vi "Update UI.vi"(7 "This VI":refnum<vi>, 8 "error in (no error)":errorcluster, 11 "Application in":refnum<class "Application.lvclass">) -> (0 "error out":errorcluster, 1 "Time":u32, 3 "Application out":refnum<class "Application.lvclass">)   [LabVIEW 2021, in "Application.lvclass"]
uses:
  Application.lvclass
  Application.lvclass/Application.ctl
  Board Game_class/Board Game.lvclass
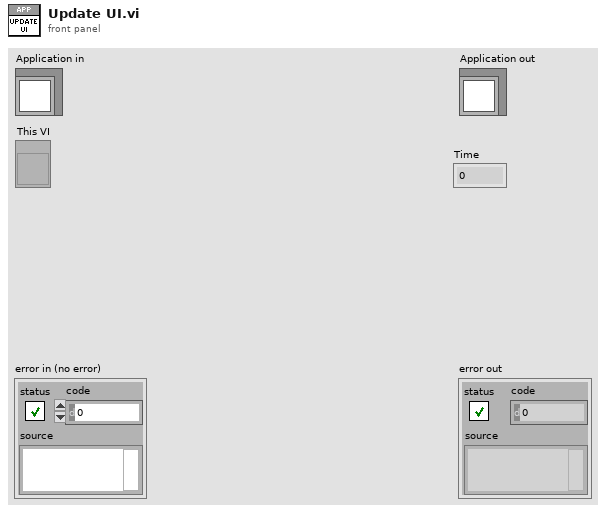
[diagram p1: front panel]
types:
  T1 = typedef "Application.lvclass/Packed Refs.ctl" = cluster{"graphics queue":refnum<queue>, "Pause Game Event":refnum<user-event>, "Stop Control Loop":refnum<user-event>, "Direction":refnum<notifier>, "play sound":refnum<user-event>, "stop sound":refnum<user-event>, "Timer":refnum<data-value>}
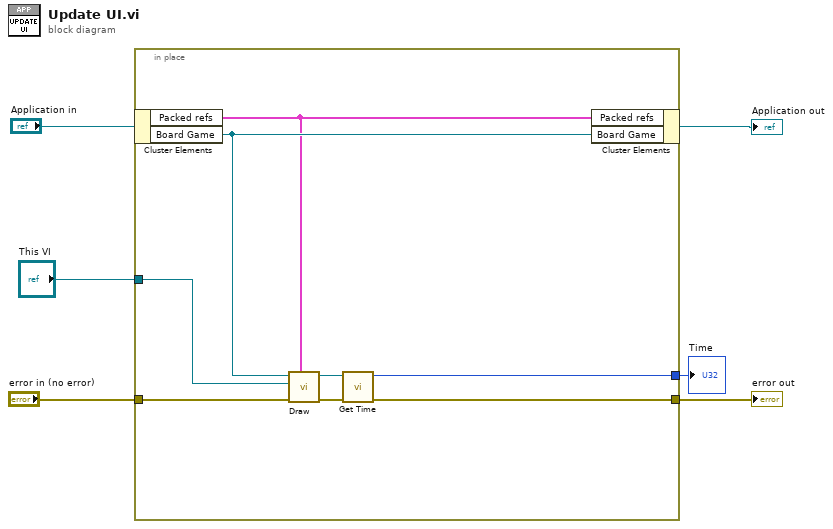
[diagram p0: block diagram]
diagram:
  n1 = in-place {
    in-place-border: "error in (no error)" -> [w13]
    in-place-border: [w11] -> w4
    in-place-border: "This VI" -> [w8]
    in-place-border: [w7] -> w1
    n2 = in-place-cluster #1("Application in") -> ("Packed refs"=w9:T1, "Board Game"=w10:refnum<class "Board Game.lvclass">)
    n3 = call "Draw.vi"("Packed refs"=w9, "error in (no error)"=w13, "This VI"=w8, "Board Game in"=w10) -> ("error out"=w12:errorcluster, "Board Game out"=w14:refnum<class "Board Game.lvclass">)  [unwired: 6 in]
    n4 = call "Get Time.vi"("error in (no error)"=w12, "Board Game in"=w14) -> ("error out"=w11:errorcluster, "Time"=w7:u32)  [unwired: 8 in]
    n5 = in-place-cluster #1("Packed refs"=w9, "Board Game"=w10) -> (→"Application out":refnum<class "Application.lvclass">)
  }
  "error out" <- w4
  "Time" <- w1
